vi "MLGet.vi"(0 "mlp in":u64, 1 "Type":i32) -> (2 "mlp out":u64, 3 "Variant":variant, 4 "Boolean":bool, 5 "Integer":i64, 6 "Real":dbl, 7 "String":string)   [LabVIEW 2014]
uses:
  LabVIEW.exe
  ml64i4.dll
  msvcrt.dll
  <vilib>/Utility/VariantDataType/VariantType.lvlib
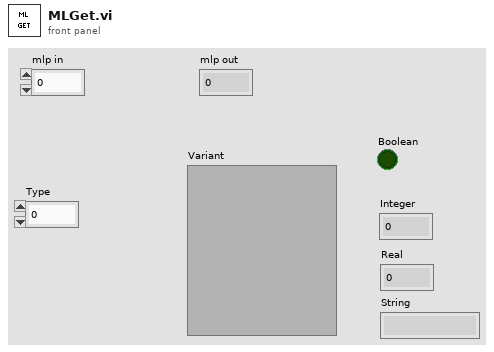
[diagram p1: front panel]
types:
  T1 = typedef "VariantType.lvlib/Type.ctl" = enum8{"Invalid Type", "Void", "I8", "I16", "I32", "I64", "U8", "U16", "U32", "U64", "Single Float", "Double Float", "Extended Float", "Single Complex", "Double Complex", "Extended Complex", "Enum U8", "Enum U16", "Enum U32", "Enum U64", "Single Float With Unit", "Double Float With Unit", "Extended Float With Unit", "Single Complex with Unit", "Double Complex with Unit", "Extended Complex with Unit", "Boolean", "String", "Path", "Picture", "Tag", "Array", "Cluster", "Variant", "LV Variant", "Waveform", "Timestamp", "Digital Waveform", "Digital Data", "ExpressData", "Refnum", "External Data", "VI", "Poly VI", "LabVIEW Class Instance", "Fixed Point"}
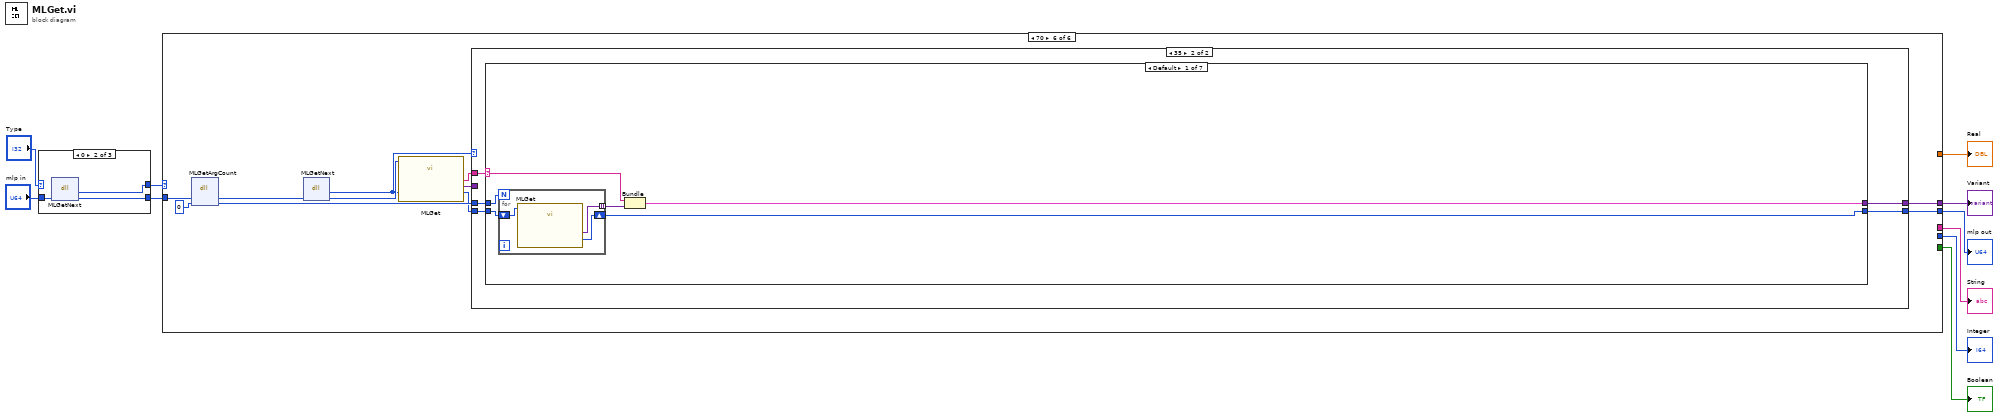
[diagram p0: block diagram]
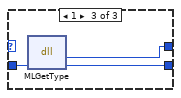
[diagram p3: hidden frame]
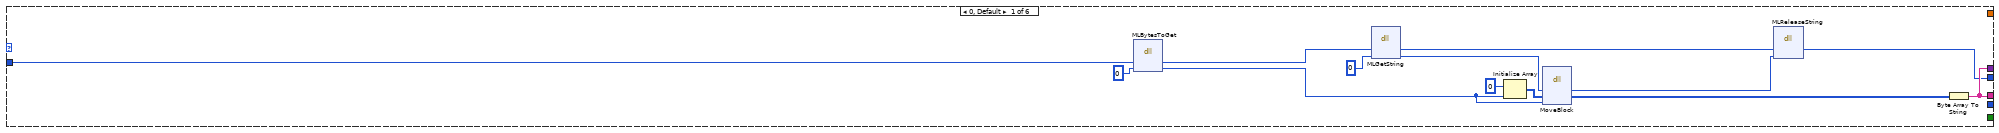
[diagram p4: hidden frame]
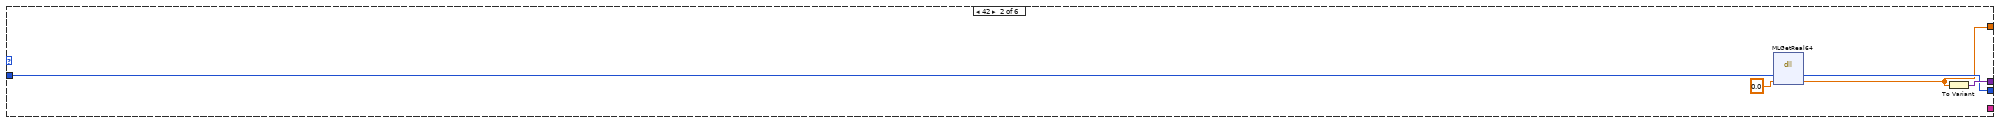
[diagram p5: hidden frame]
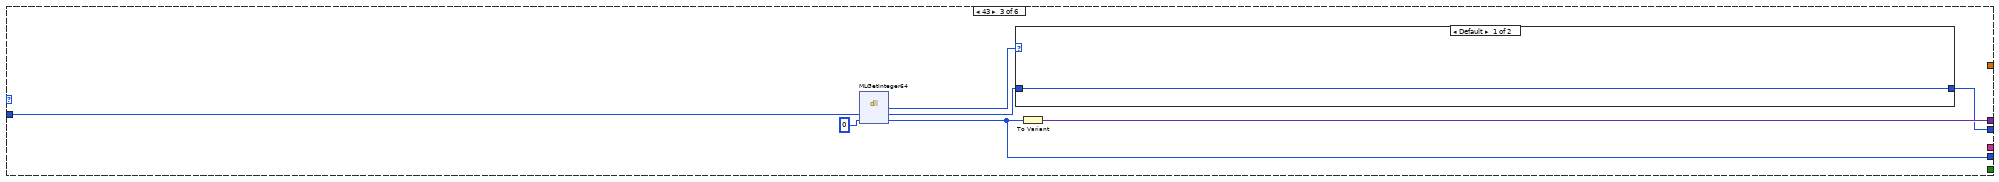
[diagram p6: hidden frame]
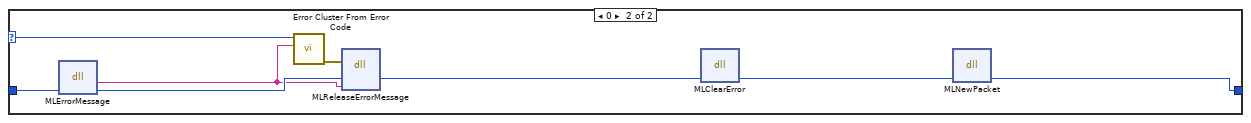
[diagram p7: hidden frame]
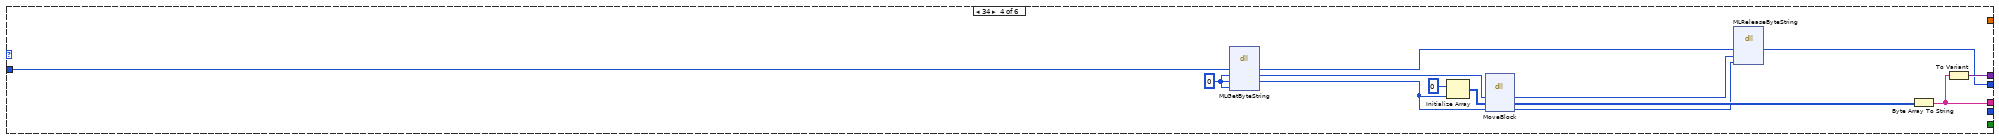
[diagram p8: hidden frame]
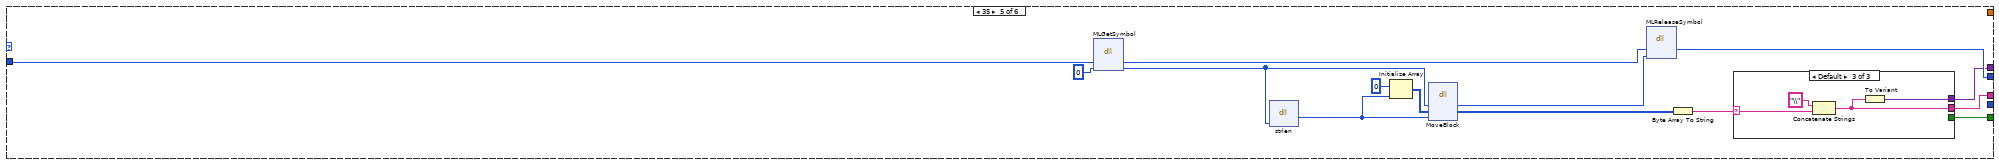
[diagram p9: hidden frame]
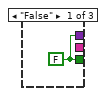
[diagram p10: hidden frame]
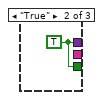
[diagram p11: hidden frame]
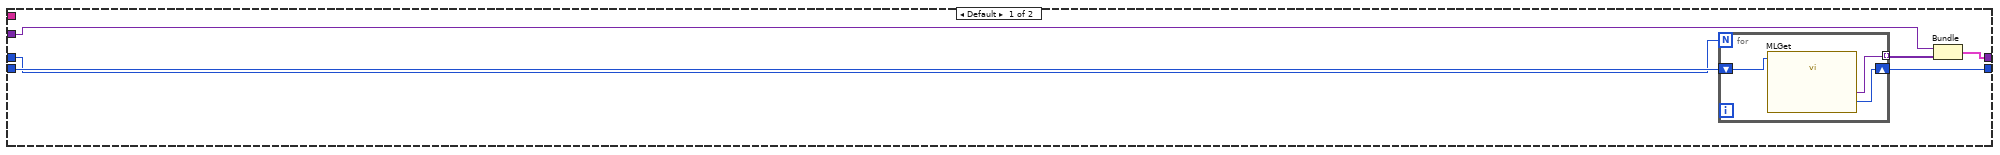
[diagram p12: hidden frame]
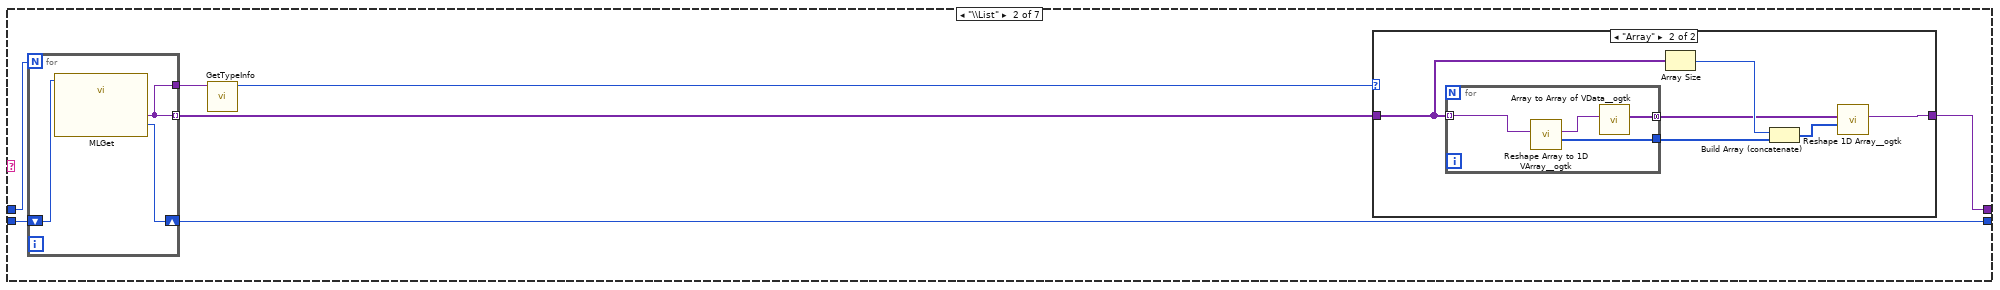
[diagram p13: hidden frame]
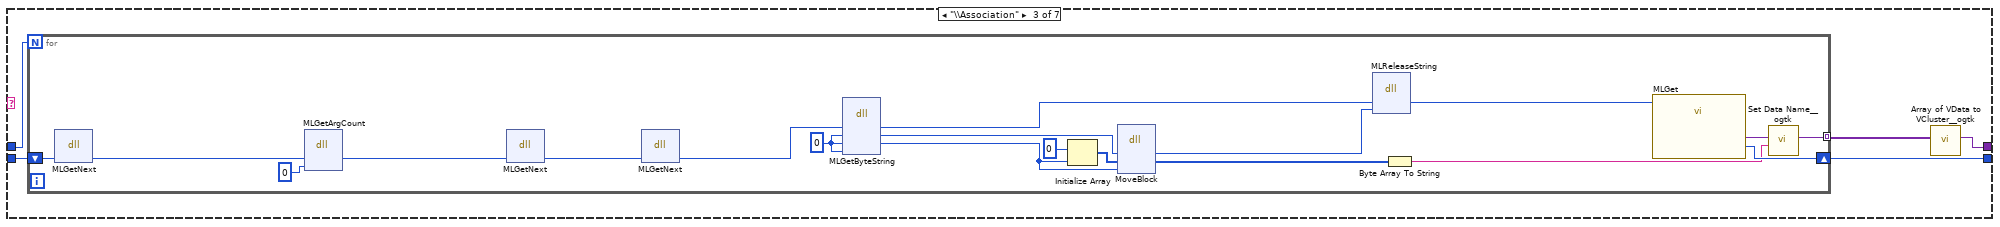
[diagram p15: hidden frame]
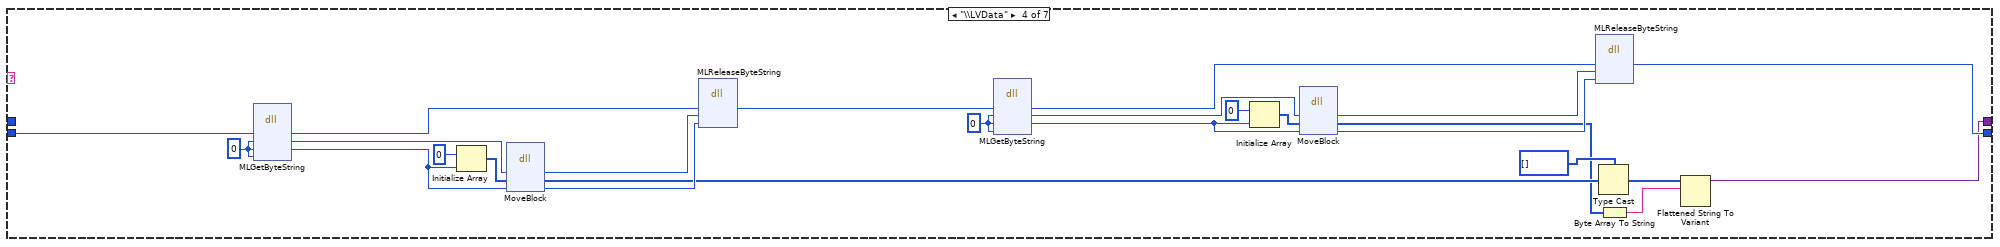
[diagram p16: hidden frame]
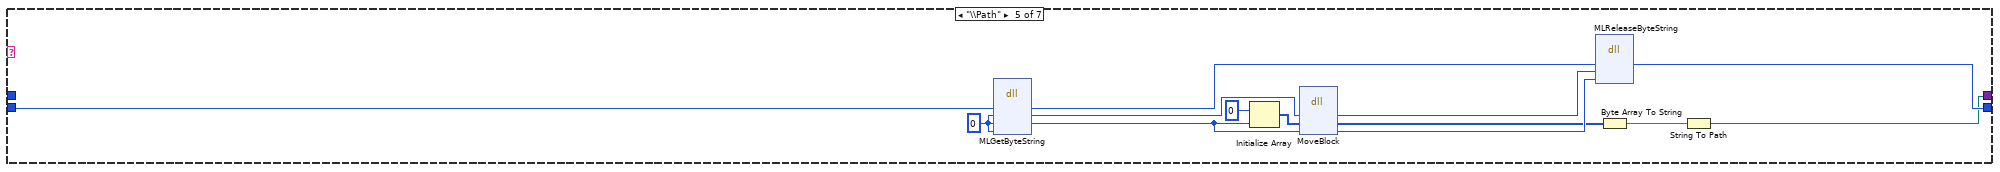
[diagram p17: hidden frame]
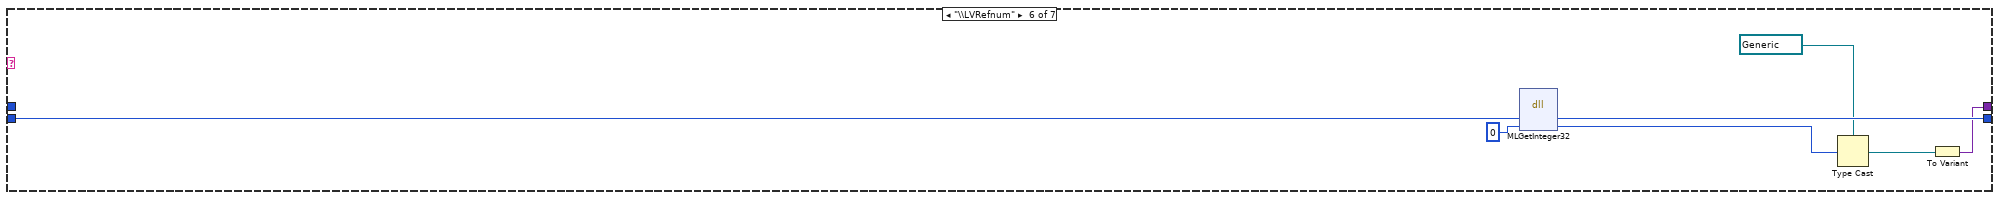
[diagram p18: hidden frame]
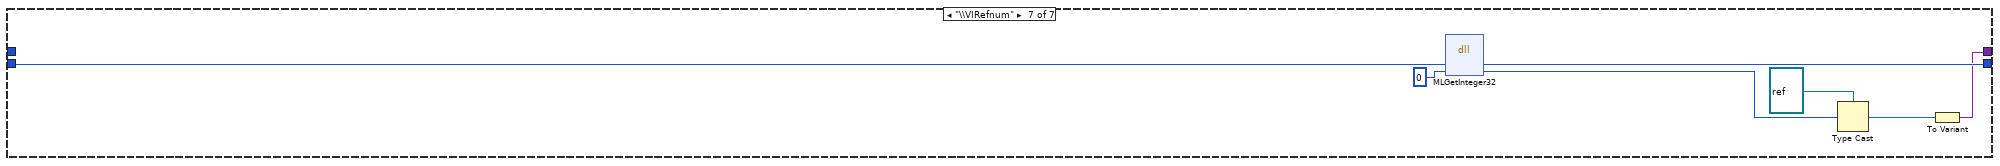
[diagram p19: hidden frame]
diagram:
  n1 = case shown="0" "Type" {
    selector: "Type" -> [w12 _ _]
    tunnel: "mlp in" -> [w11 w15 w18]
    tunnel: [w12 w14 w17] -> w5
    tunnel: [w11 w13 w16] -> w4
    frame Default {
    }
    frame 0 {
      n2 = dll-call lib="ml64i4.dll" fn="MLGetNext"("mlp"=w15) -> (w14:i32, "mlp"=w13:u64)  [unwired: 3 in, 2 out]
    }
    frame 1 {
      n3 = dll-call lib="ml64i4.dll" fn="MLGetType"("mlp"=w18) -> (w17:i32, "mlp"=w16:u64)  [unwired: 3 in, 2 out]
    }
  }
  n4 = case shown="70" w5 {
    tunnel: [w30 w36 w43 w65 w68 w93] -> w10
    tunnel: [_ w32 _ _ _ _] -> w9
    tunnel: [w30 _ _ w61 w66 _] -> w8
    tunnel: [w29 w33 w37 w55 w73 w91] -> w7
    tunnel: w4 -> [w31 w35 w42 w60 w76 w96]
    tunnel: [_ _ w40 _ _ _] -> w3
    tunnel: [_ _ _ _ w67 _] -> w2
    frame 0, Default {
      n5 = dll-call lib="ml64i4.dll" fn="MLBytesToGet"("mlp"=w31, "lenp"=0) -> ("mlp"=w23:u64, "lenp"=w25:i32)  [unwired: 4 in, 2 out]
      n6 = dll-call lib="ml64i4.dll" fn="MLGetString"("mlp"=w23, "bufp"=u64 0) -> ("mlp"=w20:u64, "bufp"=w22:u64)  [unwired: 4 in, 2 out]
      n7 = Initialize Array(u8 0 ("element"), w25) -> (w26:u8[])
      n8 = dll-call lib="LabVIEW.exe" fn="MoveBlock"("src"=w22, "dest"=w26, "size"=w25) -> ("src"=w21:u64, "dest"=w19:u8[])  [unwired: 5 in, 2 out]
      n9 = dll-call lib="ml64i4.dll" fn="MLReleaseString"("mlp"=w20, "buf"=w21) -> ("mlp"=w29:u64)  [unwired: 5 in, 2 out]
      n10 = Byte Array To String(unsigned byte array=w19) -> (string=w30:string)
    }
    frame 42 {
      n11 = dll-call lib="ml64i4.dll" fn="MLGetReal64"("mlp"=w35, "dp"=0.0) -> ("mlp"=w33:u64, "dp"=w32:dbl)  [unwired: 4 in, 2 out]
      n12 = To Variant(anything=w32) -> (Variant=w36:variant)
    }
    frame 43 {
      n13 = dll-call lib="ml64i4.dll" fn="MLGetInteger64"("mlp"=w42, "wp"=i64 0) -> (w39:i32, "mlp"=w38:u64, "wp"=w40:i64)  [unwired: 3 in, 2 out]
      n14 = case shown="Default" w39 {
        selector: w39 -> [_ w49]
        tunnel: w38 -> [w44 w51]
        tunnel: [w44 w50] -> w37
        frame Default {
        }
        frame 0 {
          n15 = dll-call lib="ml64i4.dll" fn="MLErrorMessage"("mlp"=w51) -> (w46:string, "mlp"=w48:u64)  [unwired: 3 in, 2 out]
          n16 = call <vilib>:"Error Cluster From Error Code.vi"("error message (\"\")"=w46, "error code (0)"=w49) -> ("error out"=w47:errorcluster)  [unwired: 7 in]
          n17 = dll-call lib="ml64i4.dll" fn="MLReleaseErrorMessage"(error in=w47, "mlp"=w48, "msg"=w46) -> ("mlp"=w45:u64)  [unwired: 4 in, 2 out]
          n18 = dll-call lib="ml64i4.dll" fn="MLClearError"("mlp"=w45) -> ("mlp"=w52:u64)  [unwired: 4 in, 2 out]
          n19 = dll-call lib="ml64i4.dll" fn="MLNewPacket"("mlp"=w52) -> ("mlp"=w50:u64)  [unwired: 4 in, 2 out]
        }
      }
      n20 = To Variant(anything=w40) -> (Variant=w43:variant)
    }
    frame 34 {
      w59 = 0 ("len")
      n21 = dll-call lib="ml64i4.dll" fn="MLGetByteString"("mlp"=w60, "bufp"=w59, "lenp"=w59, "missing"=w59) -> ("mlp"=w56:u64, "bufp"=w58:u64, "lenp"=w57:i32)  [unwired: 5 in, 2 out]
      n22 = Initialize Array(u8 0 ("element"), w57) -> (w63:u8[])
      n23 = dll-call lib="LabVIEW.exe" fn="MoveBlock"("src"=w58, "dest"=w63, "size"=w57) -> ("src"=w54:u64, "dest"=w62:u8[], "size"=w53:i32)  [unwired: 4 in, 2 out]
      n24 = dll-call lib="ml64i4.dll" fn="MLReleaseByteString"("mlp"=w56, "buf"=w54, "len"=w53) -> ("mlp"=w55:u64)  [unwired: 6 in, 2 out]
      n25 = Byte Array To String(unsigned byte array=w62) -> (string=w61:string)
      n26 = To Variant(anything=w61) -> (Variant=w65:variant)
    }
    frame 35 {
      n27 = dll-call lib="ml64i4.dll" fn="MLGetSymbol"("mlp"=w76, "buf"=0 ("len")) -> ("mlp"=w74:u64, "buf"=w71:u64)  [unwired: 4 in, 2 out]
      n28 = dll-call lib="msvcrt.dll" fn="strlen"("buf"=w71) -> (w70:i32)  [unwired: 4 in, 2 out]
      n29 = Initialize Array(u8 0 ("element"), w70) -> (w78:u8[])
      n30 = dll-call lib="LabVIEW.exe" fn="MoveBlock"("src"=w71, "dest"=w78, "size"=w70) -> ("src"=w72:u64, "dest"=w77:u8[])  [unwired: 5 in, 2 out]
      n31 = dll-call lib="ml64i4.dll" fn="MLReleaseSymbol"("mlp"=w74, "buf"=w72) -> ("mlp"=w73:u64)  [unwired: 5 in, 2 out]
      n32 = Byte Array To String(unsigned byte array=w77) -> (string=w69:string)
      n33 = case shown="Default" w69 {
        selector: w69 -> [_ _ w84]
        tunnel: [w80 w81 w85] -> w68
        tunnel: [w80 w81 _] -> w67
        tunnel: [_ _ w82] -> w66
        frame "False" {
          w80 = FALSE
        }
        frame "True" {
          w81 = TRUE
        }
        frame Default {
          n34 = Concatenate Strings("\\" ("string"), w84) -> (w82:string)
          n35 = To Variant(anything=w82) -> (Variant=w85:variant)
        }
      }
    }
    frame 70 {
      n36 = dll-call lib="ml64i4.dll" fn="MLGetArgCount"("mlp"=w96, "countp"=0) -> ("mlp"=w88:u64, "countp"=w90:i32)  [unwired: 4 in, 2 out]
      n37 = dll-call lib="ml64i4.dll" fn="MLGetNext"("mlp"=w88) -> (w86:i32, "mlp"=w87:u64)  [unwired: 3 in, 2 out]
      n38 = call "MLGet.vi"("mlp in"=w87, "Type"=w86) -> ("mlp out"=w89:u64, "Variant"=w92:variant, "String"=w94:string)  [unwired: 3 out]
      n39 = case shown="35" w86 {
        tunnel: w94 -> [_ w110]
        tunnel: w90 -> [w100 w109]
        tunnel: w89 -> [w102 w108]
        tunnel: [w97 w107] -> w93
        tunnel: w92 -> [w99 _]
        tunnel: [w101 w106] -> w91
        frame Default {
          n40 = for {
            N: w100 -> [_]
            shift-right: [w104] -> w101
            shift-left: w102 -> [w105]
            tunnel: [w103] -> w98 mode=indexing
            n41 = call "MLGet.vi"("mlp in"=w105) -> ("mlp out"=w104:u64, "Variant"=w103:variant)  [unwired: 1 in, 4 out]
          }
          n42 = Bundle("Variant"=w99, w98) -> (w97:cluster{"Variant":variant, variant[]})  [unwired: 1 in]
        }
        frame 35 {
          n43 = case shown="Default" w110 {
            selector: w110 -> [w113 _ _ _ _ _ _]
            tunnel: w109 -> [w114 w124 w143 _ _ _ _]
            tunnel: w108 -> [w116 w126 w145 w181 w193 w209 w216]
            tunnel: [w111 w121 w141 w165 w190 w203 w211] -> w107
            tunnel: [w115 w125 w144 w171 w191 w208 w215] -> w106
            frame Default {
              n44 = for {
                N: w114 -> [_]
                shift-right: [w118] -> w115
                shift-left: w116 -> [w119]
                tunnel: [w117] -> w112 mode=indexing
                n45 = call "MLGet.vi"("mlp in"=w119) -> ("mlp out"=w118:u64, "Variant"=w117:variant)  [unwired: 1 in, 4 out]
              }
              n46 = Bundle(w113, w112) -> (w111:cluster{string, variant[]})  [unwired: 1 in]
            }
            frame "\\List" {
              n47 = for {
                N: w124 -> [_]
                shift-right: [w139] -> w125
                shift-left: w126 -> [w140]
                tunnel: [w138] -> w122 mode=indexing
                tunnel: [w138] -> w120
                n48 = call "MLGet.vi"("mlp in"=w140) -> ("mlp out"=w139:u64, "Variant"=w138:variant)  [unwired: 1 in, 4 out]
              }
              n49 = call <vilib>:"GetTypeInfo.vi"("Variant"=w120) -> ("Type Enum"=w123:T1)  [unwired: 6 in, 4 out]
              n50 = case shown="\"Array\"" w123 {
                tunnel: w122 -> [w127 w132]
                tunnel: [w127 w130] -> w121
                frame "Invalid Type", Default {
                }
                frame "Array" {
                  n51 = for {
                    tunnel: w132 -> [w137] mode=indexing
                    tunnel: [w135] -> w133
                    tunnel: [w134] -> w128 mode=concatenating
                    n52 = call <userlib>:"Reshape Array to 1D VArray__ogtk.vi"("MultiD Array"=w137) -> ("Size(s)"=w135:u32[], "1D VArray"=w136:variant)  [unwired: 8 in, 1 out]
                    n53 = call <userlib>:"Array to Array of VData__ogtk.vi"("MultiD Array"=w136) -> ("1D Array of Variants"=w134:variant[])  [unwired: 9 in, 1 out]
                  }
                  n54 = Array Size(array=w132) -> (size(s)=w131:i32)
                  n55 = Build Array (concatenate)(w131, w133) -> (w129:u32[])
                  n56 = call <userlib>:"Reshape 1D Array__ogtk.vi"("Size(s)"=w129, "1D Array"=w128) -> ("Reshaped VArray"=w130:variant)  [unwired: 8 in, 1 out]
                }
              }
            }
            frame "\\Association" {
              n57 = for {
                N: w143 -> [_]
                shift-right: [w163] -> w144
                shift-left: w145 -> [w164]
                tunnel: [w146] -> w142 mode=indexing
                w151 = 0
                n58 = dll-call lib="ml64i4.dll" fn="MLGetNext"("mlp"=w164) -> ("mlp"=w160:u64)  [unwired: 4 in, 2 out]
                n59 = dll-call lib="ml64i4.dll" fn="MLGetArgCount"("mlp"=w160, "countp"=0) -> ("mlp"=w159:u64)  [unwired: 5 in, 2 out]
                n60 = dll-call lib="ml64i4.dll" fn="MLGetNext"("mlp"=w159) -> ("mlp"=w150:u64)  [unwired: 4 in, 2 out]
                n61 = dll-call lib="ml64i4.dll" fn="MLGetNext"("mlp"=w150) -> ("mlp"=w149:u64)  [unwired: 4 in, 2 out]
                n62 = dll-call lib="ml64i4.dll" fn="MLGetByteString"("mlp"=w149, "bufp"=w151, "lenp"=w151, "missing"=w151) -> ("mlp"=w154:u64, "bufp"=w153:u64, "lenp"=w152:i32)  [unwired: 5 in, 2 out]
                n63 = Initialize Array(u8 0 ("element"), w152) -> (w157:u8[])
                n64 = dll-call lib="LabVIEW.exe" fn="MoveBlock"("src"=w153, "dest"=w157, "size"=w152) -> ("src"=w156:u64, "dest"=w155:u8[])  [unwired: 5 in, 2 out]
                n65 = dll-call lib="ml64i4.dll" fn="MLReleaseString"("mlp"=w154, "buf"=w156) -> ("mlp"=w162:u64)  [unwired: 5 in, 2 out]
                n66 = Byte Array To String(unsigned byte array=w155) -> (string=w147:string)
                n67 = call "MLGet.vi"("mlp in"=w162) -> ("mlp out"=w163:u64, "Variant"=w148:variant)  [unwired: 1 in, 4 out]
                n68 = call <userlib>:"Set Data Name__ogtk.vi"("Data Name"=w147, "Data"=w148) -> ("Renamed Data"=w146:variant)  [unwired: 8 in, 1 out]
              }
              n69 = call <userlib>:"Array of VData to VCluster__ogtk.vi"("Array"=w142) -> ("VCluster"=w141:variant)  [unwired: 9 in, 1 out]
            }
            frame "\\LVData" {
              w178 = 0 ("len")
              w187 = 0 ("len")
              n70 = dll-call lib="ml64i4.dll" fn="MLGetByteString"("mlp"=w181, "bufp"=w187, "lenp"=w187, "missing"=w187) -> ("mlp"=w184:u64, "bufp"=w186:u64, "lenp"=w185:i32)  [unwired: 5 in, 2 out]
              n71 = Initialize Array(u8 0 ("element"), w185) -> (w188:u8[])
              n72 = dll-call lib="LabVIEW.exe" fn="MoveBlock"("src"=w186, "dest"=w188, "size"=w185) -> ("src"=w183:u64, "dest"=w167:u8[], "size"=w182:i32)  [unwired: 4 in, 2 out]
              n73 = dll-call lib="ml64i4.dll" fn="MLReleaseByteString"("mlp"=w184, "buf"=w183, "len"=w182) -> ("mlp"=w172:u64)  [unwired: 6 in, 2 out]
              n74 = dll-call lib="ml64i4.dll" fn="MLGetByteString"("mlp"=w172, "bufp"=w178, "lenp"=w178, "missing"=w178) -> ("mlp"=w175:u64, "bufp"=w177:u64, "lenp"=w176:i32)  [unwired: 5 in, 2 out]
              n75 = Initialize Array(u8 0 ("element"), w176) -> (w179:u8[])
              n76 = dll-call lib="LabVIEW.exe" fn="MoveBlock"("src"=w177, "dest"=w179, "size"=w176) -> ("src"=w174:u64, "dest"=w166:u8[], "size"=w173:i32)  [unwired: 4 in, 2 out]
              n77 = dll-call lib="ml64i4.dll" fn="MLReleaseByteString"("mlp"=w175, "buf"=w174, "len"=w173) -> ("mlp"=w171:u64)  [unwired: 6 in, 2 out]
              n78 = Type Cast(type=i16[] [] ("type string"), x=w167) -> (*(type *) &x=w168:i16[])
              n79 = Byte Array To String(unsigned byte array=w166) -> (string=w170:string)
              n80 = Flattened String To Variant(6:w170, 7:w168) -> (3:w165:variant)  [unwired: 1 in, 1 out]
            }
            frame "\\Path" {
              w199 = 0 ("len")
              n81 = dll-call lib="ml64i4.dll" fn="MLGetByteString"("mlp"=w193, "bufp"=w199, "lenp"=w199, "missing"=w199) -> ("mlp"=w196:u64, "bufp"=w198:u64, "lenp"=w197:i32)  [unwired: 5 in, 2 out]
              n82 = Initialize Array(u8 0 ("element"), w197) -> (w200:u8[])
              n83 = dll-call lib="LabVIEW.exe" fn="MoveBlock"("src"=w198, "dest"=w200, "size"=w197) -> ("src"=w195:u64, "dest"=w192:u8[], "size"=w194:i32)  [unwired: 4 in, 2 out]
              n84 = dll-call lib="ml64i4.dll" fn="MLReleaseByteString"("mlp"=w196, "buf"=w195, "len"=w194) -> ("mlp"=w191:u64)  [unwired: 6 in, 2 out]
              n85 = Byte Array To String(unsigned byte array=w192) -> (string=w202:string)
              n86 = String To Path(string=w202) -> (path=w190:path)
            }
            frame "\\LVRefnum" {
              n87 = dll-call lib="ml64i4.dll" fn="MLGetInteger32"("mlp"=w209, "ip"=u32 0) -> ("mlp"=w208:u64, "ip"=w205:u32)  [unwired: 4 in, 2 out]
              n88 = Type Cast(type=refnum<vi> refnum ("reference"), x=w205) -> (*(type *) &x=w206:refnum<vi>)
              n89 = To Variant(anything=w206) -> (Variant=w203:variant)
            }
            frame "\\VIRefnum" {
              n90 = dll-call lib="ml64i4.dll" fn="MLGetInteger32"("mlp"=w216, "ip"=u32 0) -> ("mlp"=w215:u64, "ip"=w213:u32)  [unwired: 4 in, 2 out]
              n91 = Type Cast(type=refnum<vi> refnum ("vi reference"), x=w213) -> (*(type *) &x=w214:refnum<vi>)
              n92 = To Variant(anything=w214) -> (Variant=w211:variant)
            }
          }
        }
      }
    }
  }
  "Variant" <- w10
  "Real" <- w9
  "String" <- w8
  "mlp out" <- w7
  "Integer" <- w3
  "Boolean" <- w2
